vi "Init Events.vi"(8 "error in (no error)":errorcluster, 11 "LV Client in":refnum<class "LV Client.lvclass">) -> (0 "error out":errorcluster, 3 "LV Client out":refnum<class "LV Client.lvclass">)   [LabVIEW 2020, in "LV Client.lvclass"]
uses:
  LV Client.lvclass
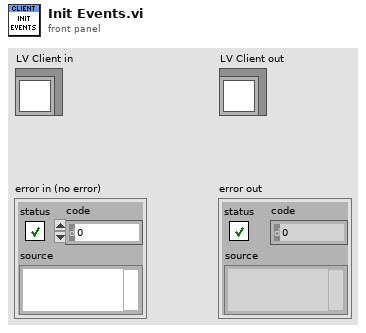
[diagram p1: front panel]
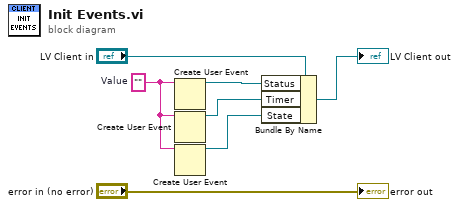
[diagram p0: block diagram]
diagram:
  w6 = ""  # Value
  n1 = Create User Event(user event datatype=w6) -> (user event=w4:refnum<user-event>)  [unwired: 1 in, 1 out]
  n2 = Create User Event(user event datatype=w6) -> (user event=w5:refnum<user-event>)  [unwired: 1 in, 1 out]
  n3 = Create User Event(user event datatype=w6) -> (user event=w3:refnum<user-event>)  [unwired: 1 in, 1 out]
  n4 = Bundle By Name(cluster="LV Client in", "Status"=w4, "Timer"=w5, "State"=w3) -> (→"LV Client out":refnum<class "LV Client.lvclass">)
  "error out" <- "error in (no error)"
